vi "core_query_error_code_database.vi"(10 "code in":i32) -> (1 "code description":string, 2 "code out":i32)   [LabVIEW 2015]
uses:
  core_is_code_plus_eco.vi
  core_pm_global_eco.vi
  polys/poly_global_eco_plus.vi
  polys/poly_global_eco_minus.vi
  core_global_ECO.vi
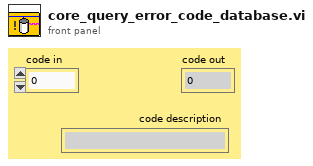
[diagram p1: front panel]
types:
  T1 = enum16{"open", "replace", "create", "open or create", "replace or create", "replace or create with confirmation"}
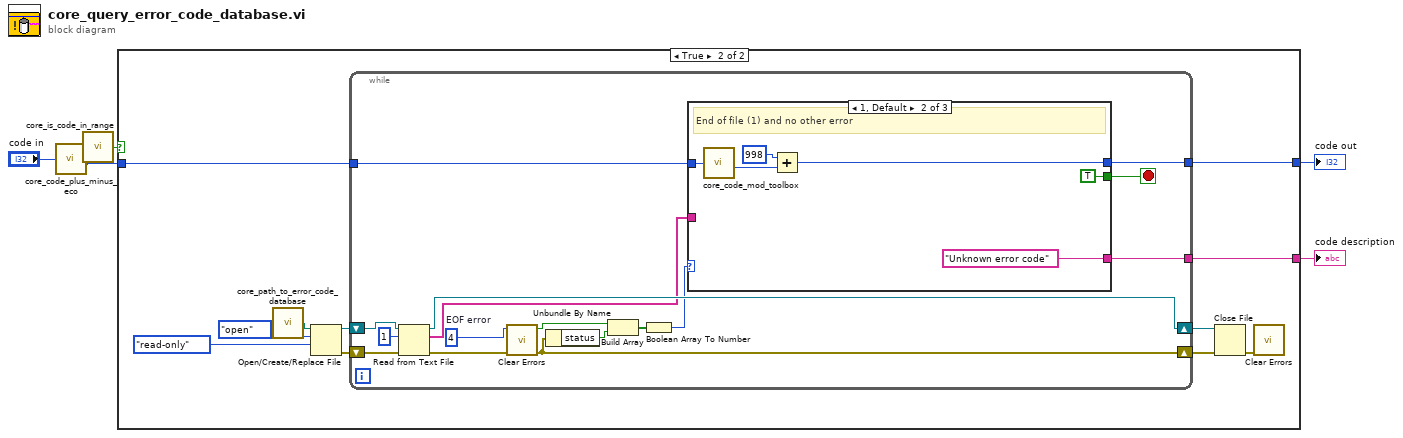
[diagram p0: block diagram]
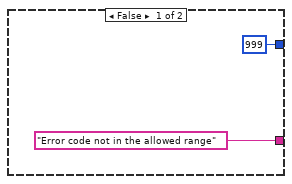
[diagram p2: hidden frame]
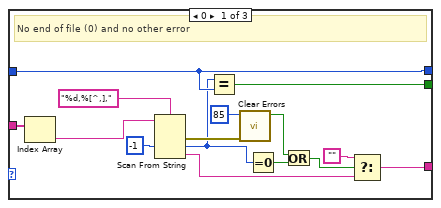
[diagram p3: hidden frame]
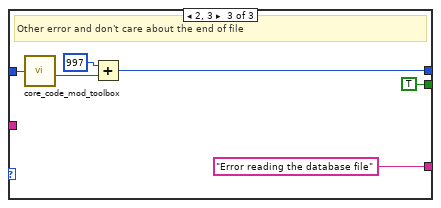
[diagram p4: hidden frame]
diagram:
  n1 = call "core_code_plus_minus_eco.vi"("code in"="code in") -> ("code w/out ECO"=w1:i32)  [unwired: 8 in, 1 out]
  n2 = call "core_is_code_in_range.vi"("code (w/out ECO)"=w1) -> ("code in allowed range?"=w2:bool)  [unwired: 4 in]
  n3 = case shown="True" w2 {
    tunnel: w1 -> [_ w12]
    tunnel: ["Error code not in the allowed range" w10] -> w4
    tunnel: [999 ("code w/out ECO") w9] -> w3
    frame False {
    }
    frame True {
      n4 = call "core_path_to_error_code_database.vi"() -> ("path to database"=w8:path)
      n5 = Open/Create/Replace File(file path (use dialog)=w8, operation (0:open)=T1."open", access (0:read/write)=enum16{"read/write", "read-only", "write-only"}."read-only") -> (refnum out=w18:refnum<file>, error out=w17:errorcluster)  [unwired: 3 in, 1 out]
      n6 = while {
        shift-right: [w33] -> w16
        shift-left: w18 -> [w34]
        tunnel: [w27] -> w10
        shift-right: [w25] -> w15
        shift-left: w17 -> [w32]
        tunnel: [w26] -> w9
        tunnel: w12 -> [w19]
        stop <- w20 stop-if-true
        w28 = 4  # EOF error
        n7 = Read from Text File(file (use dialog)=w34, count=1, error in=w32) -> (refnum out=w33:refnum<file>, text=w30:string[], error out=w29:errorcluster)  [unwired: 1 in, 1 out]
        n8 = call <vilib>:"Clear Errors.vi"("error in (no error)"=w29, "specific error code to clear (0: all)"=w28) -> ("error out"=w25:errorcluster, "specific error cleared?"=w21:bool)  [unwired: 4 in]
        n9 = Unbundle By Name(w25) -> ("status"=w24:bool)
        n10 = Build Array(w21, w24) -> (w23:bool[])
        n11 = Boolean Array To Number(Boolean array=w23) -> (number=w22:u32)
        n12 = case shown="1, Default" w22 {
          tunnel: w30 -> [w49 _ _]
          tunnel: [w40 "Unknown error code" "Error reading the database file"] -> w27
          tunnel: [w43 TRUE TRUE] -> w20
          tunnel: [w42 w52 w60] -> w26
          tunnel: w19 -> [w42 w51 w57]
          frame 0 {
            # "No end of file (0) and no other error"
            n13 = Index Array(array=w49) -> (element=w48:string)  [unwired: 1 in]
            n14 = Scan From String(format string="%d,%[^,],", input string=w48, default 1=-1 ("default value 1")) -> (error out=w46:errorcluster, output 1=w41:i32, output 2=w35:string)  [unwired: 3 in, 2 out]
            n15 = Equal?(x=w41, y=w42) -> (x = y?=w43:bool)
            n16 = call <vilib>:"Clear Errors.vi"("error in (no error)"=w46, "specific error code to clear (0: all)"=85) -> ("specific error cleared?"=w39:bool)  [unwired: 4 in, 1 out]
            n17 = Equal To 0?(x=w41) -> (x = 0?=w38:bool)
            n18 = Or(x=w39, y=w38) -> (x .or. y?=w37:bool)
            n19 = Select(t="", s=w37, f=w35) -> (s? t:f=w40:string)
          }
          frame 1, Default {
            # "End of file (1) and no other error"
            n20 = call "core_code_mod_toolbox.vi"("error code"=w51) -> ("toolbox offset"=w50:i32)  [unwired: 8 in, 1 out]
            n21 = Add(x=998, y=w50) -> (x+y=w52:i32)
          }
          frame 2, 3 {
            # "Other error and don't care about the end of file"
            n22 = call "core_code_mod_toolbox.vi"("error code"=w57) -> ("toolbox offset"=w56:i32)  [unwired: 8 in, 1 out]
            n23 = Add(x=997, y=w56) -> (x+y=w60:i32)
          }
        }
      }
      n24 = Close File(refnum=w16, error in=w15) -> (error out=w11:errorcluster)  [unwired: 1 out]
      n25 = call <vilib>:"Clear Errors.vi"("error in (no error)"=w11) -> ()  [unwired: 5 in, 2 out]
    }
  }
  "code description" <- w4
  "code out" <- w3
